vi "ADC AI Global (Avg).vi"() -> ()   [LabVIEW 2013]
panel:
  out "AI22-47 (Avg)":fxp<+/-,28,17>[](array[numeric])
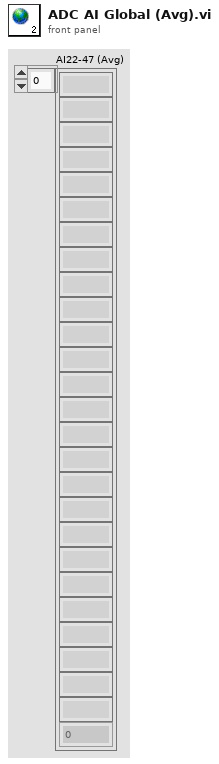
[diagram p1: front panel]
diagram:
